vi "Resize.Screen Coordinates at X,Y Distance from the Origin.vi"(5 "Y Units (Percent)":enum16{"Percent", "Pixels"}(ring), 6 "Origin (Top Left)":T1(ring), 7 "X Units (Percent)":enum16{"Percent", "Pixels"}(ring), 8 "error in (no error)":errorcluster, 9 "Y Distance":dbl=1.0, 10 "X Distance":dbl=1.0, 11 "Pane Reference":refnum<vi>) -> (0 "error out":errorcluster, 1 "Screen Y Coordinate":dbl, 2 "Screen X Coordinate":dbl)   [LabVIEW 2024, in "EQMF.lvlib" / "Controls.lvlib"]
uses:
  Controls.lvlib
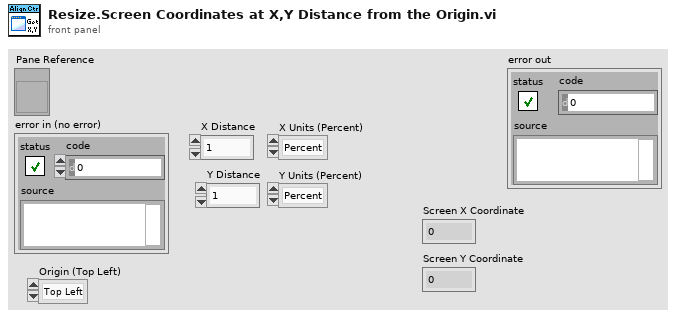
[diagram p1: front panel]
types:
  T1 = enum16{"Top Left", "Bottom Right", "Top Right", "Bottom Left"}
  T2 = typedef "LVRectTypeDef.ctl" = cluster{"Left":i16, "Top":i16, "Right":i16, "Bottom":i16}
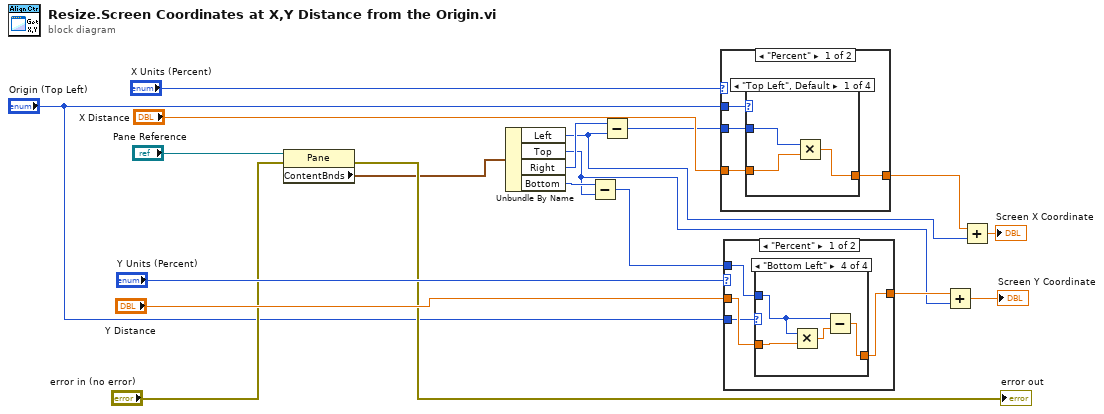
[diagram p0: block diagram]
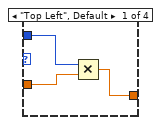
[diagram p2: hidden frame]
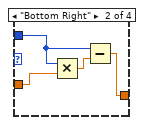
[diagram p3: hidden frame]
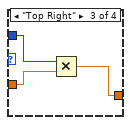
[diagram p4: hidden frame]
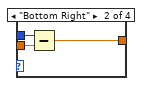
[diagram p6: hidden frame]
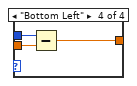
[diagram p8: hidden frame]
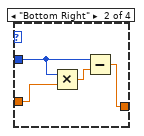
[diagram p9: hidden frame]
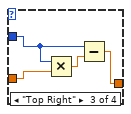
[diagram p10: hidden frame]
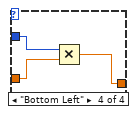
[diagram p11: hidden frame]
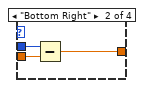
[diagram p13: hidden frame]
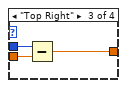
[diagram p14: hidden frame]
diagram:
  n1 = property class="Pane"(reference="Pane Reference", error in="error in (no error)") -> (error out=→"error out":errorcluster, "ContentBnds"=w8:T2)  [unwired: 1 out]
  n2 = Unbundle By Name(w8) -> ("Left"=w3:i16, "Top"=w2:i16, "Right"=w7:i16, "Bottom"=w6:i16)
  n3 = Subtract(x=w6, y=w2) -> (x-y=w4:i16)
  n4 = Subtract(x=w7, y=w3) -> (x-y=w5:i16)
  n5 = case shown="\"Percent\"" "X Units (Percent)" {
    tunnel: "X Distance" -> [w22 w40]
    tunnel: w5 -> [w21 w41]
    tunnel: [w23 w39] -> w10
    tunnel: "Origin (Top Left)" -> [w20 w38]
    frame "Percent" {
      n6 = case shown="\"Top Left\", Default" w20 {
        tunnel: [w26 w28 w31 w35] -> w23
        tunnel: w22 -> [w25 w30 w32 w36]
        tunnel: w21 -> [w24 w27 w33 w37]
        frame "Top Left", Default {
          n7 = Multiply(x=w24, y=w25) -> (x*y=w26:dbl)
        }
        frame "Bottom Right" {
          n8 = Multiply(x=w27, y=w30) -> (x*y=w29:dbl)
          n9 = Subtract(x=w27, y=w29) -> (x-y=w28:dbl)
        }
        frame "Top Right" {
          n10 = Multiply(x=w33, y=w32) -> (x*y=w34:dbl)
          n11 = Subtract(x=w33, y=w34) -> (x-y=w31:dbl)
        }
        frame "Bottom Left" {
          n12 = Multiply(x=w37, y=w36) -> (x*y=w35:dbl)
        }
      }
    }
    frame "Pixels" {
      n13 = case shown="\"Top Left\", Default" w38 {
        tunnel: w41 -> [_ w45 w48 _]
        tunnel: w40 -> [w42 w44 w47 w49]
        tunnel: [w42 w43 w46 w49] -> w39
        frame "Top Left", Default {
        }
        frame "Bottom Right" {
          n14 = Subtract(x=w45, y=w44) -> (x-y=w43:dbl)
        }
        frame "Top Right" {
          n15 = Subtract(x=w48, y=w47) -> (x-y=w46:dbl)
        }
        frame "Bottom Left" {
        }
      }
    }
  }
  n16 = case shown="\"Percent\"" "Y Units (Percent)" {
    tunnel: "Y Distance" -> [w53 w70]
    tunnel: w4 -> [w52 w71]
    tunnel: [w50 w69] -> w9
    tunnel: "Origin (Top Left)" -> [w51 w68]
    frame "Percent" {
      n17 = case shown="\"Bottom Left\"" w51 {
        tunnel: [w56 w58 w61 w64] -> w50
        tunnel: w53 -> [w55 w60 w62 w65]
        tunnel: w52 -> [w54 w57 w63 w66]
        frame "Top Left", Default {
          n18 = Multiply(x=w54, y=w55) -> (x*y=w56:dbl)
        }
        frame "Bottom Right" {
          n19 = Multiply(x=w57, y=w60) -> (x*y=w59:dbl)
          n20 = Subtract(x=w57, y=w59) -> (x-y=w58:dbl)
        }
        frame "Top Right" {
          n21 = Multiply(x=w63, y=w62) -> (x*y=w61:dbl)
        }
        frame "Bottom Left" {
          n22 = Multiply(x=w66, y=w65) -> (x*y=w67:dbl)
          n23 = Subtract(x=w66, y=w67) -> (x-y=w64:dbl)
        }
      }
    }
    frame "Pixels" {
      n24 = case shown="\"Top Left\", Default" w68 {
        tunnel: w71 -> [_ w75 _ w79]
        tunnel: w70 -> [w72 w74 w76 w78]
        tunnel: [w72 w73 w76 w77] -> w69
        frame "Top Left", Default {
        }
        frame "Bottom Right" {
          n25 = Subtract(x=w75, y=w74) -> (x-y=w73:dbl)
        }
        frame "Top Right" {
        }
        frame "Bottom Left" {
          n26 = Subtract(x=w79, y=w78) -> (x-y=w77:dbl)
        }
      }
    }
  }
  n27 = Add(x=w9, y=w2) -> (x+y=→"Screen Y Coordinate":dbl)
  n28 = Add(x=w10, y=w3) -> (x+y=→"Screen X Coordinate":dbl)
